vi "Handle Double Click on Element.vi"(8 "error in (no error)":errorcluster, 10 "Unique ID":string, 11 "Test Executive Builder in":refnum<class "Test Executive Builder.lvclass">) -> (0 "error out":errorcluster, 3 "Test Executive Builder out":refnum<class "Test Executive Builder.lvclass">)   [LabVIEW 2017, in "Test Executive Builder.lvclass"]
uses:
  Test Executive Builder.lvclass
  Source/Test Executive Builder Model/Test Executive Builder Model/Test Executive Builder Model.lvclass
  C:/Users/jonmc/Documents/Git/Test Executive Builder/Source/Test Executive Builder Model/Test Executive Builder Model/Test Executive Builder Model.lvclass
  4765e24f-05e7-406f-ac83-caaf36ff0286.vi
  Source/Test Executive Builder Dialogs/ITest Executive Builder Dialog/ITest Executive Builder Dialog.lvclass
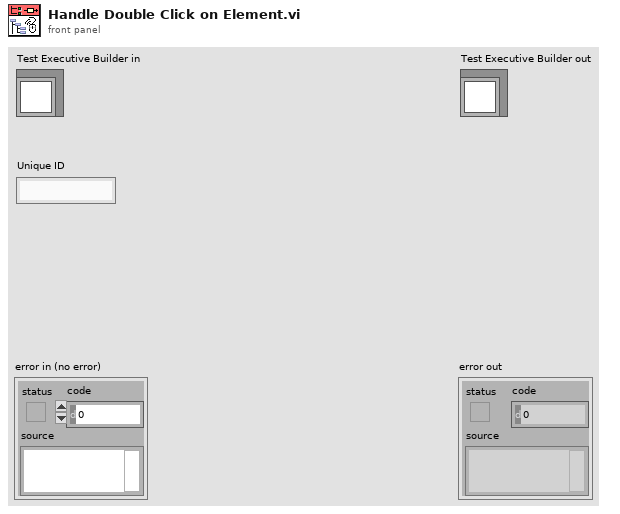
[diagram p1: front panel]
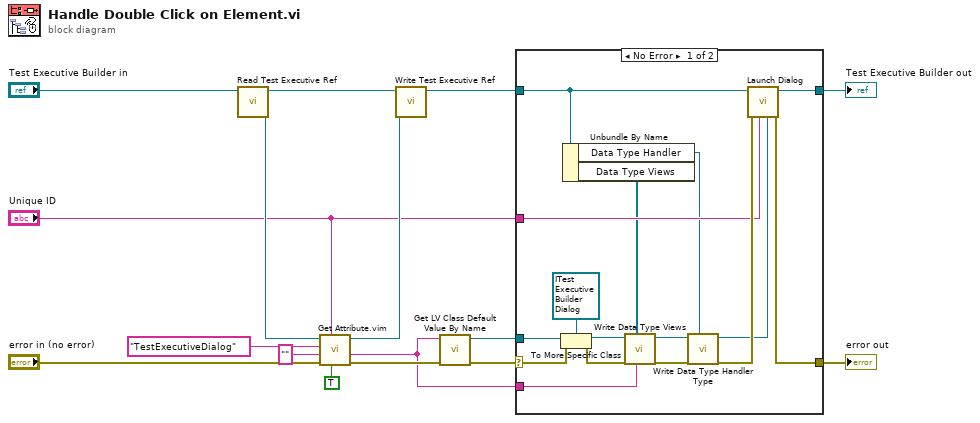
[diagram p0: block diagram]
diagram:
  n1 = call "Read Test Executive Ref.vi"("Test Executive Builder Model in"="Test Executive Builder in") -> ("Test Executive Ref"=w13:refnum<data-value>, "Test Executive Builder Model out"=w15:refnum<class "Test Executive Builder.lvclass">)  [unwired: 9 in]
  n2 = call "Get Attribute.vim"("Include Private?"=TRUE, "ID"="Unique ID", "error in (no error)"="error in (no error)", "Type"="", "Attribute Name"="TestExecutiveDialog", "Test Executive Ref"=w13) -> ("error out"=w8:errorcluster, "Attribute"=w1:string, "Test Executive Ref out"=w12:refnum<data-value>)  [unwired: 1 in, 2 out]
  n3 = call "Write Test Executive Ref.vi"("Test Executive Ref"=w12, "Test Executive Builder Model in"=w15) -> ("Test Executive Builder Model out"=w5:refnum<class "Test Executive Builder.lvclass">)  [unwired: 9 in]
  n4 = call <vilib>:"Get LV Class Default Value By Name.vi"("error in (no error)"=w8, "class name"=w1) -> ("error out"=w6:errorcluster, "object"=w7:refnum<class>)  [unwired: 8 in]
  n5 = case shown="No Error" w6 {
    selector: w6 -> [w29 _]
    tunnel: w7 -> [w30 _]
    tunnel: w5 -> [w22 w31]
    tunnel: [w27 w31] -> w4
    tunnel: [w25 _] -> w3
    tunnel: "Unique ID" -> [w24 _]
    tunnel: w1 -> [w20 _]
    frame No Error {
      n6 = To More Specific Class(target class=refnum<class "ITest Executive Builder Dialog.lvclass"> refnum ("ITest Executive Builder Dialog.lvclass"), reference=w30, error in=w29) -> (specific class reference=w23:refnum<class "ITest Executive Builder Dialog.lvclass">, error out=w26:errorcluster)
      n7 = Unbundle By Name(w22) -> ("Data Type Handler"=w17:refnum<class "Test Executive Builder Data Type Handler.lvclass">, "Data Type Views"=w21:refnum<class "IAttribute Data Type View.lvclass">[])
      n8 = call "Write Data Type Views.vi"("Popup Title"=w20, "Data Type Views"=w21, "ITest Executive Builder Dialog in"=w23) -> ("ITest Executive Builder Dialog out"=w19:refnum<class "ITest Executive Builder Dialog.lvclass">)  [unwired: 8 in]
      n9 = call "Write Data Type Handler Type.vi"("Data Type Handler"=w17, "ITest Executive Builder Dialog in"=w19) -> ("ITest Executive Builder Dialog out"=w18:refnum<class "ITest Executive Builder Dialog.lvclass">)  [unwired: 9 in]
      n10 = call "Launch Dialog.vi"("Dialog Type"=w18, "Unique ID"=w24, "error in (no error)"=w26, "Test Executive Builder in"=w22) -> ("error out"=w25:errorcluster, "Test Executive Builder out"=w27:refnum<class "Test Executive Builder.lvclass">)  [unwired: 6 in]
    }
    frame Error {
    }
  }
  "error out" <- w3
  "Test Executive Builder out" <- w4
